vi "open Serial MB.vi"(7 "Slave ID":u8=1, 8 "Error in":errorcluster caption="Error in (no error)", 9 "Serial Config":T1={"baud rate (bps)"=115200, "stop bits"=10, "parity"=0, "flow control"=0, "timeout"=1000, "retries"=1} {"stop bits" items=["1.0"=10, "1.5"=15, "2.0"=20]; "parity" items=["None", "Odd", "Even", "Mark", "Space"]; "flow control" items=["None", "XON/XOFF", "RTS/CTS", "XON/XOFF & RTS/CTS", "DTR/DSR", "XON/XOFF & DTR/DSR"]}, 10 "VISA Resource":refnum<visa-resource-name>, 11 "MB session in":refnum<class "MB_Master.lvclass">) -> (0 "error out":errorcluster, 3 "MB session out":refnum<class "MB_Master.lvclass">)   [LabVIEW 2016, in "环境动力监测库.lvlib" / "UPS库.lvlib"]
uses:
  <vilib>/Plasmionique/MB Master/MB_Master/MB_Master.lvclass
  <vilib>/Plasmionique/MB Master/MB_Master_Serial/MB_Master_Serial.lvclass
  C:/Program Files (x86)/National Instruments/LabVIEW 2016/vi.lib/Plasmionique/MB Master/MB_Master/MB_Master.lvclass
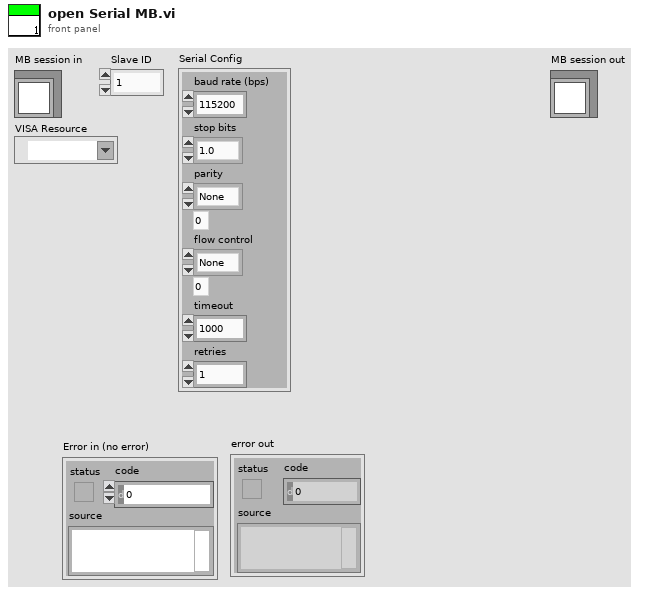
[diagram p1: front panel]
types:
  T1 = cluster{"baud rate (bps)":u32, "stop bits":u16, "parity":u16, "flow control":u16, "timeout":u32, "retries":i32}
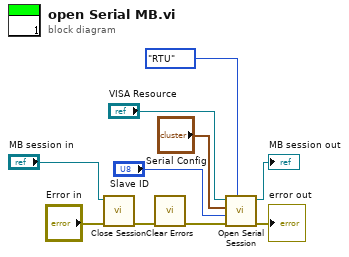
[diagram p0: block diagram]
diagram:
  n1 = call-dynamic "Close Session.vi"("error in (no error)"="Error in", "MB session in"="MB session in") -> ("error out"=w8:errorcluster)  [unwired: 9 in]
  n2 = call <vilib>:"Clear Errors.vi"("error in (no error)"=w8) -> ("error out"=w7:errorcluster)  [unwired: 5 in, 1 out]
  n3 = call <vilib>:"Open Serial Session.vi"("Mode (RTU)"=enum16{"RTU", "ASCII"}."RTU", "Error in"=w7, "Slave ID"="Slave ID", "Serial Config"="Serial Config", "VISA Resource"="VISA Resource") -> ("Error out"=→"error out":errorcluster, "MB_Serial session"=→"MB session out":refnum<class "MB_Master_Serial.lvclass">)  [unwired: 5 in]
